vi "Enable-disable DIO Bits For Jog Mode.vi"(4 "error in (no error)":errorcluster, 5 "Enable DIO bits (disable)":bool, 6 "Axis (1)":i32=1 min=1 max=3, 7 "VISA resource name":refnum<visa-resource-name>) -> (0 "error out":errorcluster, 3 "VISA resource name out":refnum<visa-resource-name>)   [LabVIEW 2015, in "Newport ESP301.lvlib"]
doc: "This command is used to disable or enable jogging of a requested axis through DIO bits."
uses:
  Newport ESP301.lvlib
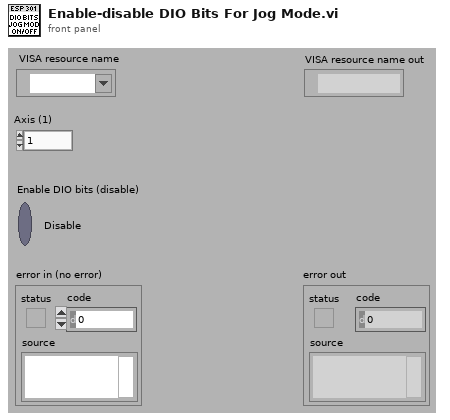
[diagram p1: front panel]
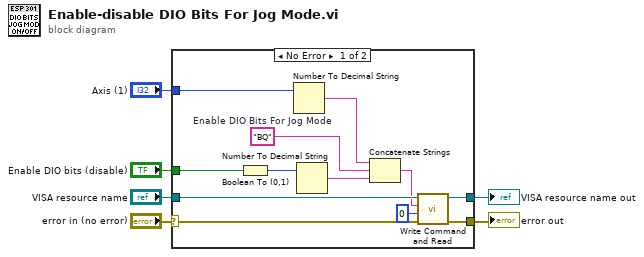
[diagram p0: block diagram]
diagram:
  n1 = case shown="No Error" "error in (no error)" {
    selector: "error in (no error)" -> [w17 w20]
    tunnel: [w16 w20] -> w6
    tunnel: "VISA resource name" -> [w18 w19]
    tunnel: [w15 w19] -> w5
    tunnel: "Axis (1)" -> [w10 _]
    tunnel: "Enable DIO bits (disable)" -> [w8 _]
    frame No Error {
      w11 = "BQ"  # Enable DIO Bits For Jog Mode
      n2 = Boolean To (0,1)(Boolean=w8) -> (0, 1=w13:i16)
      n3 = Number To Decimal String(number=w10) -> (decimal integer string=w14:string)  [unwired: 1 in]
      n4 = Number To Decimal String(number=w13) -> (decimal integer string=w12:string)  [unwired: 1 in]
      n5 = Concatenate Strings(w14, w11, w12) -> (w9:string)
      n6 = call "Write Command and Read.vi"("error in (no error)"=w17, "Bytes to read (100)"=u32 0, "Command"=w9, "VISA resource name"=w18) -> ("error out"=w16:errorcluster, "VISA resource name out"=w15:refnum<visa-resource-name>)  [unwired: 3 in, 1 out]
    }
    frame Error {
    }
  }
  "error out" <- w6
  "VISA resource name out" <- w5
